vi "readCurrent_Sensor.vi"(8 "error in (no error)":errorcluster) -> (0 "error out":errorcluster)   [LabVIEW 2013]
uses:
  My Computer/Controls/Sensors State.ctl
  <vilib>/myRIO/Instrument Drivers/Onboard IO/AI/vis/Smart Open.vi
  <vilib>/myRIO/Instrument Drivers/Onboard IO/AI/vis/Read.vi
  <vilib>/myRIO/Instrument Drivers/Onboard IO/AI/vis/Open.vi
  <vilib>/myRIO/Common/Instrument Driver Framework/myRIO v1.0/AI/vis/myRIO v1.1 Open AI.vi
  <vilib>/myRIO/Common/Instrument Driver Framework/Utilities/vis/Validate Channels.vi
  <vilib>/myRIO/Common/Instrument Driver Framework/myRIO v1.0/AI/vis/myRIO v1.0 Reserve AI.vi
  <vilib>/myRIO/Common/Instrument Driver Framework/myRIO v1.0/AI/vis/myRIO v1.0 Build MUX Configuration AI.vi
  <vilib>/myRIO/Common/Instrument Driver Framework/myRIO v1.0/Resource Manager/vis/myRIO v1.0 Reserve Channel List.vi
  <vilib>/myRIO/Common/Instrument Driver Framework/myRIO v1.0/Resource Manager/vis/myRIO v1.0 Reserve Channel.vi
  <vilib>/myRIO/Common/Instrument Driver Framework/myRIO v1.0/Resource Manager/vis/myRIO v1.0 Unreserve Channel.vi
  <vilib>/myRIO/Common/Instrument Driver Framework/myRIO v1.0/Resource Manager/vis/myRIO v1.0 Build Mutex Name.vi
  <vilib>/myRIO/Common/Instrument Driver Framework/myRIO v1.0/myRIO v1.1 Open.vi
  <vilib>/myRIO/Common/Instrument Driver Framework/myRIO v1.0/AI/vis/myRIO v1.0 Get Scaling Constants AI.vi
  <vilib>/Utility/VariantDataType/GetNumericInfo.vi
  <vilib>/Utility/error.llb/Error Cluster From Error Code.vi
  <vilib>/myRIO/Common/Instrument Driver Framework/Utilities/vis/IO Manager.vi
  <vilib>/myRIO/Common/Instrument Driver Framework/Utilities/vis/Configuration Manager.vi
  <vilib>/myRIO/Common/Instrument Driver Framework/myRIO v1.0/myRIO v1.0 Close.vi
  <vilib>/myRIO/Common/Instrument Driver Framework/myRIO v1.0/AI/vis/myRIO v1.0 Read AI.vi
panel:
  out "Main Current":dbl
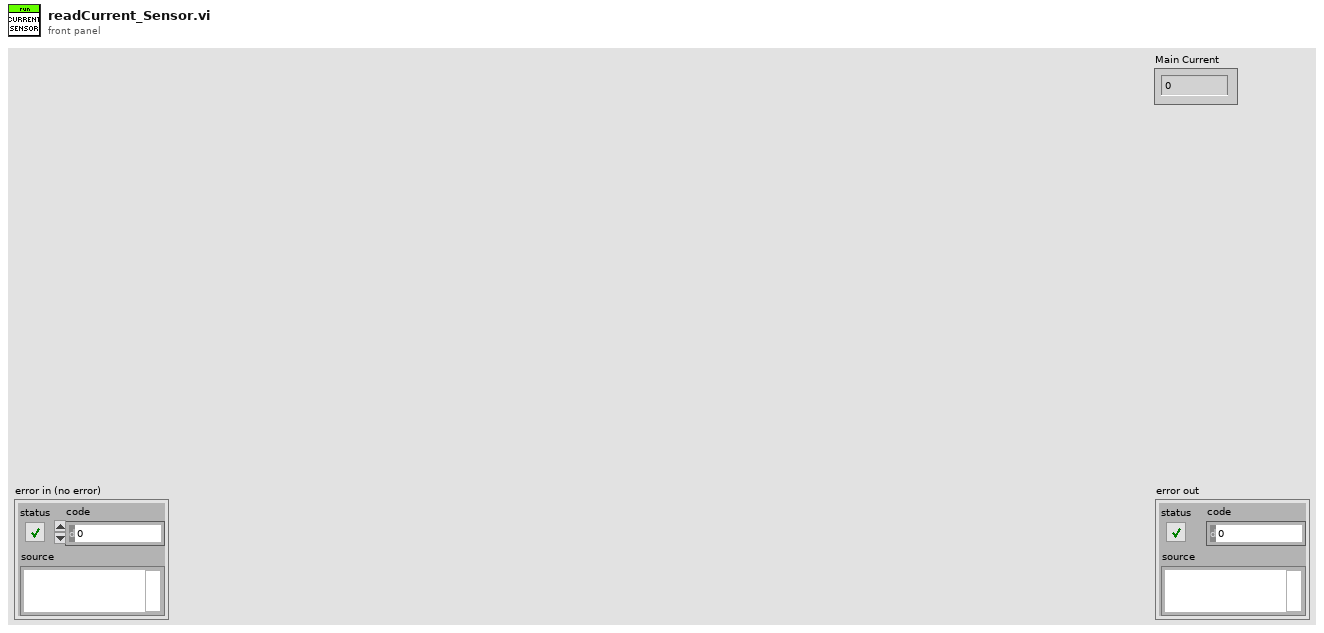
[diagram p1: front panel]
types:
  T1 = typedef "Sensors State.ctl" = cluster{"Leakage-Sensor_enabled":bool, "IMU_enabled":bool, "Swimbladder Fill-State-Sensor_enabled":bool, "Flow-Sensor_enabled":bool, "Depth-Sensor_enabled":bool, "Current-Sensor_enabled":bool, "Calibrate Depth":bool, "SB_Piston_Stuck_Detect_enabled":bool, "Check_too_Deep_enabled":bool}
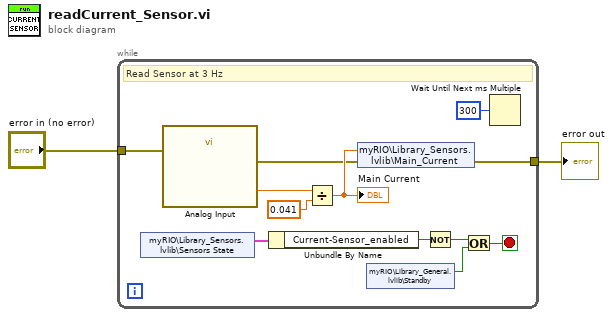
[diagram p0: block diagram]
diagram:
  n1 = while {
    tunnel: "error in (no error)" -> [w10]
    tunnel: [w5] -> w1
    stop <- w7 stop-if-true
    # "Read Sensor at 3 Hz"
    n2 = shared-variable "myRIO\\Library_Sensors.lvlib\\Sensors State"() -> (w4:T1)  [unwired: 1 in, 1 out]
    n3 = call "Analog Input"("error in (no error)"=w10) -> ("Current Voltage Drop (A/AI3 (Pin 9))"=w14:dbl, "error out"=w6:errorcluster)  [unwired: 25 in]
    n4 = Unbundle By Name(w4) -> ("Current-Sensor_enabled"=w3:bool)
    n5 = Divide(x=w14, y=0.041) -> (x/y=w12:dbl)
    "Main Current" <- w12
    n6 = shared-variable "myRIO\\Library_Sensors.lvlib\\Main_Current"(w12, error in=w6) -> (error out=w5:errorcluster)
    n7 = shared-variable "myRIO\\Library_General.lvlib\\Standby"() -> (w8:bool)  [unwired: 1 in, 1 out]
    n8 = Not(x=w3) -> (.not. x?=w9:bool)
    n9 = Or(x=w9, y=w8) -> (x .or. y?=w7:bool)
    n10 = Wait Until Next ms Multiple(millisecond multiple=u32 300) -> ()  [unwired: 1 out]
  }
  "error out" <- w1
